vi "Send LON command to SR752.vi"(8 "error in":errorcluster, 11 "TCP Network Connection in":refnum<k5>) -> (0 "error out":errorcluster, 2 "data out":string, 3 "TCP Network Connection out":refnum<k5>)   [LabVIEW 2023]
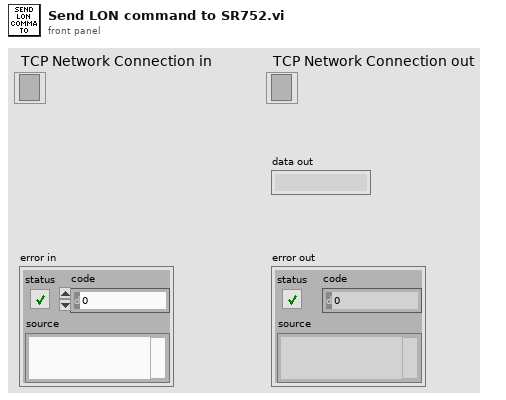
[diagram p1: front panel]
types:
  T1 = enum16{"Standard", "Buffered", "CRLF", "Immediate"}
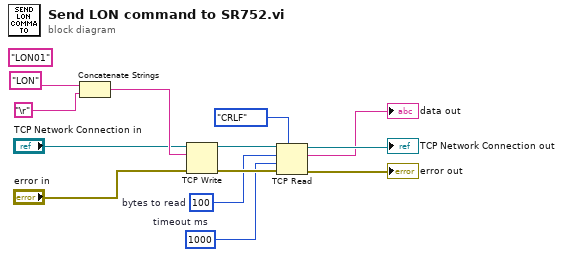
[diagram p0: block diagram]
diagram:
  (unwired) "LON01"
  w5 = 1000  # timeout ms
  w6 = 100  # bytes to read
  n1 = Concatenate Strings("LON" ("Command"), "\r") -> (w12:string)
  n2 = TCP Write(connection ID="TCP Network Connection in", data in=w12, error in (no error)="error in") -> (connection ID out=w8:refnum<k5>, error out=w7:errorcluster)  [unwired: 1 in, 1 out]
  n3 = TCP Read(connection ID=w8, bytes to read=w6, error in (no error)=w7, 7:T1."CRLF" ("mode (standard)"), 9:w5) -> (connection ID out=→"TCP Network Connection out":refnum<k5>, data out=→"data out":string, error out=→"error out":errorcluster)
